vi "sample_a1.vi"(7 "delta":i32, 9 "threshold":i32, 11 "times":i32) -> (3 "ai":sgl)   [LabVIEW 2012]
uses:
  <vilib>/eio/EIONode/EIONode.xnode
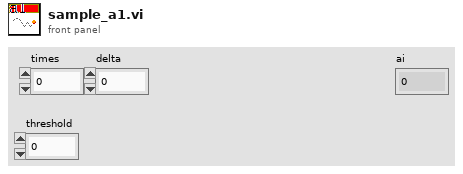
[diagram p1: front panel]
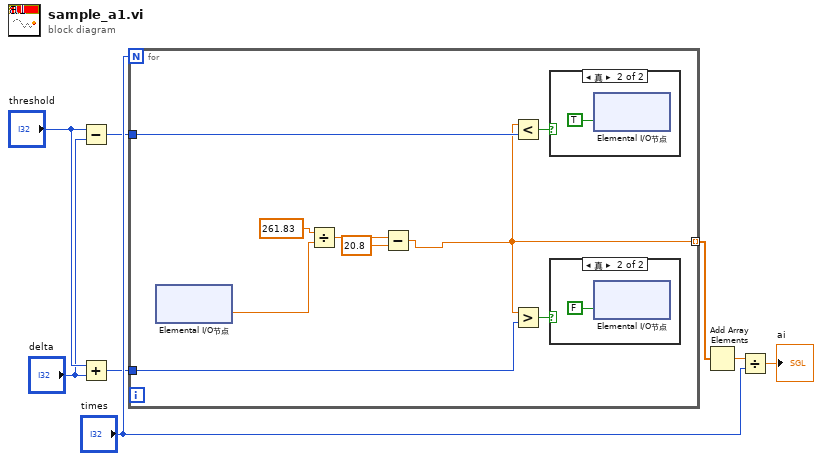
[diagram p0: block diagram]
diagram:
  n1 = Subtract(x="threshold", y="delta") -> (x-y=w3:i32)
  n2 = Add(x="threshold", y="delta") -> (x+y=w5:i32)
  n3 = for {
    N: "times" -> [_]
    tunnel: w5 -> [w17]
    tunnel: w3 -> [w16]
    tunnel: [w10] -> w1 mode=indexing
    n4 = xnode "Elemental I/O节点"() -> ("AI1"=w12:sgl)  [unwired: 1 in, 1 out]
    n5 = Divide(x=261.83 ("y"), y=w12) -> (x/y=w11:dbl)
    n6 = Subtract(x=w11, y=20.8) -> (x-y=w10:dbl)
    n7 = Less?(x=w10, y=w16) -> (x < y?=w14:bool)
    n8 = Greater?(x=w10, y=w17) -> (0:w15:bool)
    n9 = case shown="真" w14 {
      frame False {
      }
      frame True {
        n10 = xnode "Elemental I/O节点"("DIO0"=TRUE) -> ()  [unwired: 1 in, 1 out]
      }
    }
    n11 = case shown="真" w15 {
      frame False {
      }
      frame True {
        n12 = xnode "Elemental I/O节点"("DIO0"=FALSE) -> ()  [unwired: 1 in, 1 out]
      }
    }
  }
  n13 = Add Array Elements(numeric array=w1) -> (sum=w8:dbl)
  n14 = Divide(x=w8, y="times") -> (x/y=→"ai":dbl)
